vi "CreatePinmapWith3Pins_QueryPins_3PinsFound.vi"() -> (6 "pass":bool, 8 "result":string, 15 "error out":errorcluster)   [LabVIEW 2020]
uses:
  Pin Map Client_lv/Pin Map Client_v1/RPC Messages/ni_measurementlink_pinmap_v1_CreatePinMapFromXmlRequest.ctl
  Pin Map Client_lv/Pin Map Client_v1/RPC Messages/ni_measurementlink_pinmap_v1_QueryPinsRequest.ctl
  Pin Map Client_lv/Pin Map Client_v1/Pin Map Client_v1.lvlib
panel:
  # "Test assumes discovery service and pin map service has already been started."
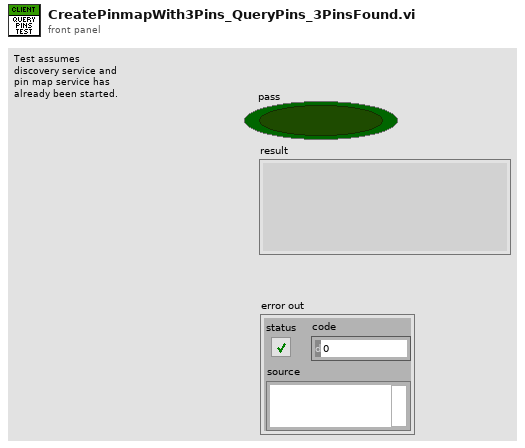
[diagram p1: front panel]
types:
  T1 = typedef "Pin Map Client_v1.lvlib/ni_measurementlink_pinmap_v1_QueryPinsRequest.ctl" = cluster{"pin_map_id":string, "instrument_type_id":string}
  T2 = typedef "Pin Map Client_v1.lvlib/ni_measurementlink_pinmap_v1_CreatePinMapFromXmlRequest.ctl" = cluster{"pin_map_id":string, "pin_map_xml":string}
  T3 = typedef "grpc-lvsupport-release.lvlib/grpcId.ctl" = u64
  T4 = typedef "Pin Map Client_v1.lvlib/ni_measurementlink_pinmap_v1_PinMap.ctl" = cluster{"pin_map_id":string}
  T5 = typedef "Pin Map Client_v1.lvlib/ni_measurementlink_pinmap_v1_QueryPinsResponse.ctl" = cluster{"pins":T6[], "pin_groups":T7[]}
  T6 = typedef "Pin Map Client_v1.lvlib/ni_measurementlink_pinmap_v1_QueryPinsResponse_PinDefinition.ctl" = cluster{"display_name":string, "is_system_pin":bool}
  T7 = typedef "Pin Map Client_v1.lvlib/ni_measurementlink_pinmap_v1_QueryPinsResponse_PinGroupDefinition.ctl" = cluster{"display_name":string, "pin_or_group_references":string[], "resolved_pins":string[]}
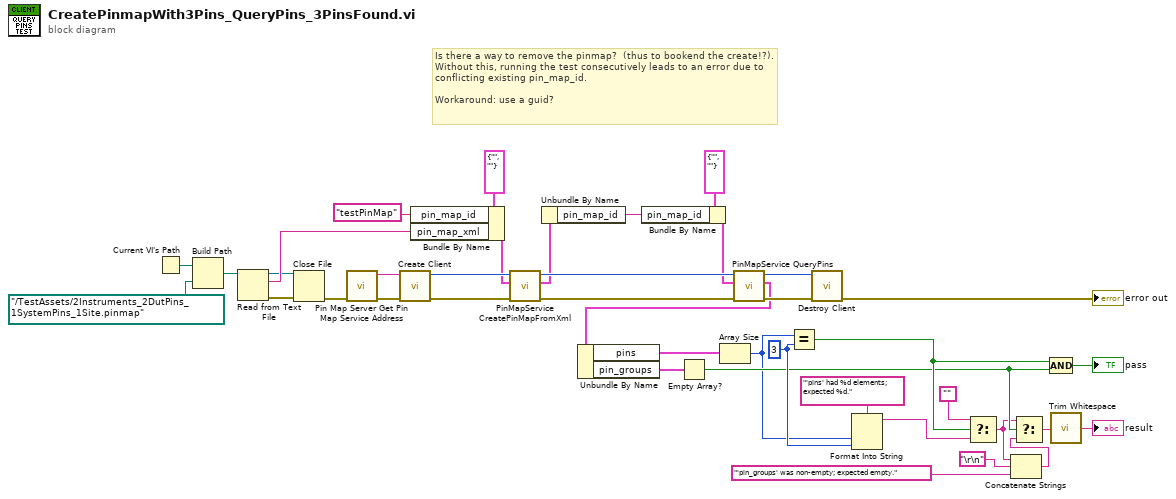
[diagram p0: block diagram]
diagram:
  w16 = 3 ("y")
  # "Is there a way to remove the pinmap?  (thus to bookend the create!?).  Without this, running the test consecutively leads to an error due to conflicting existing pin_map_id.\n\nWorkaround: use a guid?"
  n1 = Current VI's Path() -> (path=w37:path)
  n2 = Build Path(base path=w37, name or relative path=path "../TestAssets/2Instruments_2DutPins_1SystemPins_1Site.pinmap") -> (appended path=w35:path)
  n3 = Read from Text File(file (use dialog)=w35) -> (refnum out=w31:refnum<file>, text=w33:string, error out=w32:errorcluster)  [unwired: 3 in, 1 out]
  n4 = Close File(refnum=w31, error in=w32) -> (error out=w1:errorcluster)  [unwired: 1 out]
  n5 = call "Pin Map Server Get Pin Map Service Address.vi"("error in (no error)"=w1) -> ("error out"=w2:errorcluster, "address"=w3:string)  [unwired: 9 in]
  n6 = call "Create Client.vi"("error in"=w2, "address"=w3) -> ("error out"=w39:errorcluster, "gRPC ID Out"=w38:T3)  [unwired: 8 in]
  n7 = Bundle By Name(cluster=T2 {"pin_map_id"="", "pin_map_xml"=""} ("Request Data"), "pin_map_id"="testPinMap", "pin_map_xml"=w33) -> (w30:T2)
  n8 = call "PinMapService CreatePinMapFromXml.vi"("error in"=w39, "Request Data"=w30, "gRPC ID"=w38) -> ("error out"=w28:errorcluster, "Response Data"=w22:T4, "gRPC ID out"=w29:T3)  [unwired: 6 in]
  n9 = Unbundle By Name(w22) -> ("pin_map_id"=w23:string)
  n10 = Bundle By Name(cluster=T1 {"pin_map_id"="", "instrument_type_id"=""} ("Request Data"), "pin_map_id"=w23) -> (w21:T1)
  n11 = call "PinMapService QueryPins.vi"("error in"=w28, "Request Data"=w21, "gRPC ID"=w29) -> ("error out"=w27:errorcluster, "Response Data"=w20:T5, "gRPC ID out"=w26:T3)  [unwired: 6 in]
  n12 = Unbundle By Name(w20) -> ("pins"=w19:T6[], "pin_groups"=w5:T7[])
  n13 = Empty Array?(array=w5) -> (empty?=w12:bool)
  n14 = Array Size(array=w19) -> (size(s)=w4:i32)
  n15 = Equal?(x=w4, y=w16) -> (x = y?=w15:bool)
  n16 = call "Destroy Client.vi"("error in"=w27, "gRPC ID"=w26) -> ("error out"=→"error out":errorcluster)  [unwired: 9 in]
  n17 = Format Into String(format string="'pins' had %d elements; expected %d.", w4, w16) -> (resulting string=w14:string)  [unwired: 2 in, 1 out]
  n18 = Select(t="", s=w15, f=w14) -> (s? t:f=w8:string)
  n19 = Concatenate Strings(w8, "\r\n", "'pin_groups' was non-empty; expected empty.") -> (w11:string)
  n20 = Select(t=w8, s=w12, f=w11) -> (s? t:f=w7:string)
  n21 = Compound Arithmetic op=AND(w15, w12) -> (→"pass":bool)
  n22 = call <vilib>:"Trim Whitespace.vi"("string"=w7) -> ("trimmed string"=→"result":string)  [unwired: 1 in]
